vi "Dec_9 - noRamp.vi"() -> ()   [LabVIEW 2020]
uses:
  <vilib>/Utility/error.llb/DialogType.ctl
  <vilib>/Analysis/3filter.llb/Filter Passband Type.ctl
  <vilib>/DAQmx/read.llb/DAQmx Read (Analog 1D DBL NChan 1Samp).vi
  <vilib>/DAQmx/create/channels.llb/DAQmx Create Channel (AI-Voltage-Basic).vi
  <vilib>/DAQmx/configure/timing.llb/DAQmx Timing (Sample Clock).vi
  <vilib>/DAQmx/miscellaneous.llb/DAQmx Fill In Error Info.vi
  <vilib>/Analysis/3filter.llb/Butterworth Filter (DBL).vi
  <vilib>/Utility/file.llb/Write Delimited Spreadsheet (string).vi
  <vilib>/Utility/file.llb/Write Delimited Spreadsheet (DBL).vi
  <vilib>/Analysis/NI_AALBase.lvlib
panel:
  out "Actual Swing":bool
  out "N° step Max":i32
  in  "Choose Automatic Mode":string(combo)
  in  "START":bool
  out "Step Number":i32
  out "Step Counted":bool
  out "Time to Peak (sec)":dbl=200.0
  out "Swing ON Time (sec)":dbl
  in  "Only pre-tension load":bool
  out "Gyro":dynamicdata(graph)
  out "Max Square Wave duration (sec)":dbl
  out "Swing Start Time (sec)":dbl
  out "Time Saved":bool
  out "Pre-Tension Load (N)":dbl
  out "Target Load (N)":dbl=2.0
  out "Release":bool
  out "Pull":bool
  in  "Working Mode":string(combo)
  out "Load Cell":dbl
  in  "Pull CMD":bool
  in  "Release CMD":bool
  out "Load Cell":dynamicdata(graph)
  in  "Motor Torque":dbl(slide) scale=0.0..5.0
  in  "Master Stop":bool
  out "Consumer Loop Speed (ms)":u32
  out "Producer Loop Speed (ms)":u32
  out "Swing":bool
  out "Force Plate":dynamicdata(graph)
  out "Accelerometers":dynamicdata(graph)
  out "Enlapsed Time (sec)":dbl
  # "Choose work mode"
  # "Manual"
  # "Automatic"
  # "Ramp Between-Step Mode"
  # "Ramp Within-Step Mode"
  # "Indicators"
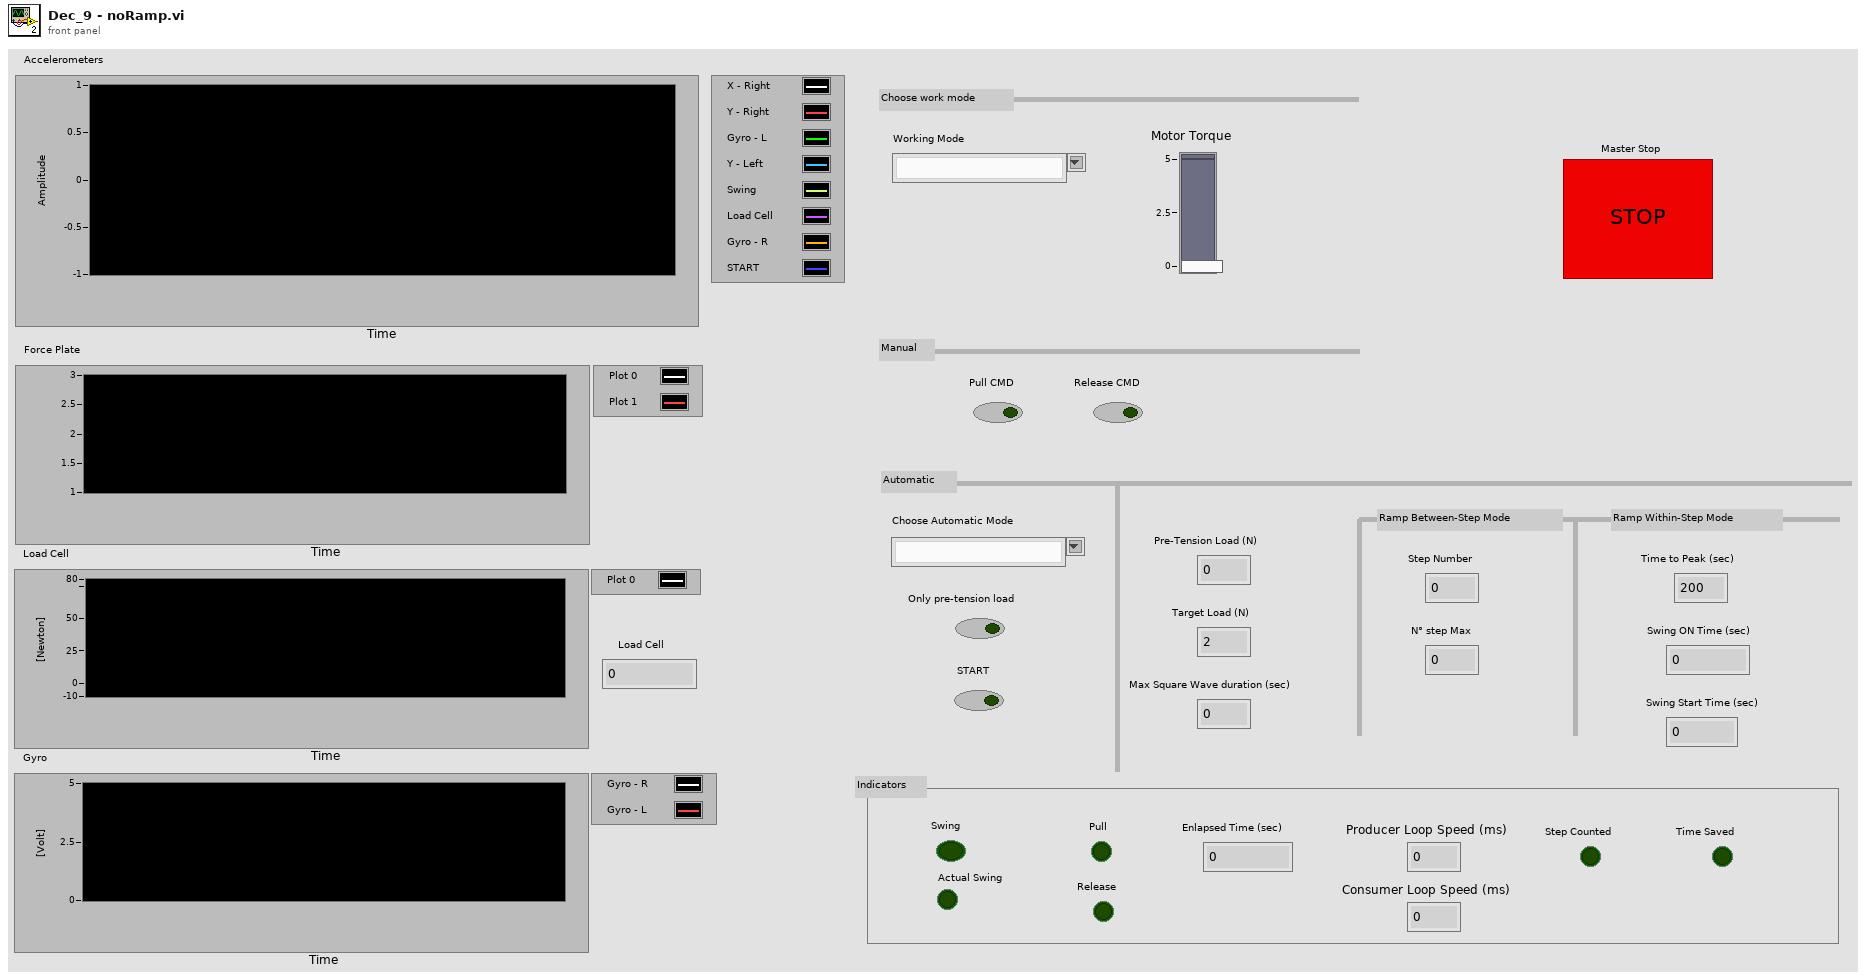
[diagram p1: front panel]
types:
  T1 = typedef "DialogType.ctl" = u16
  T2 = typedef "NI_AALBase.lvlib/Filter Passband Type.ctl" = enum32{"Lowpass", "Highpass", "Bandpass", "Bandstop"}
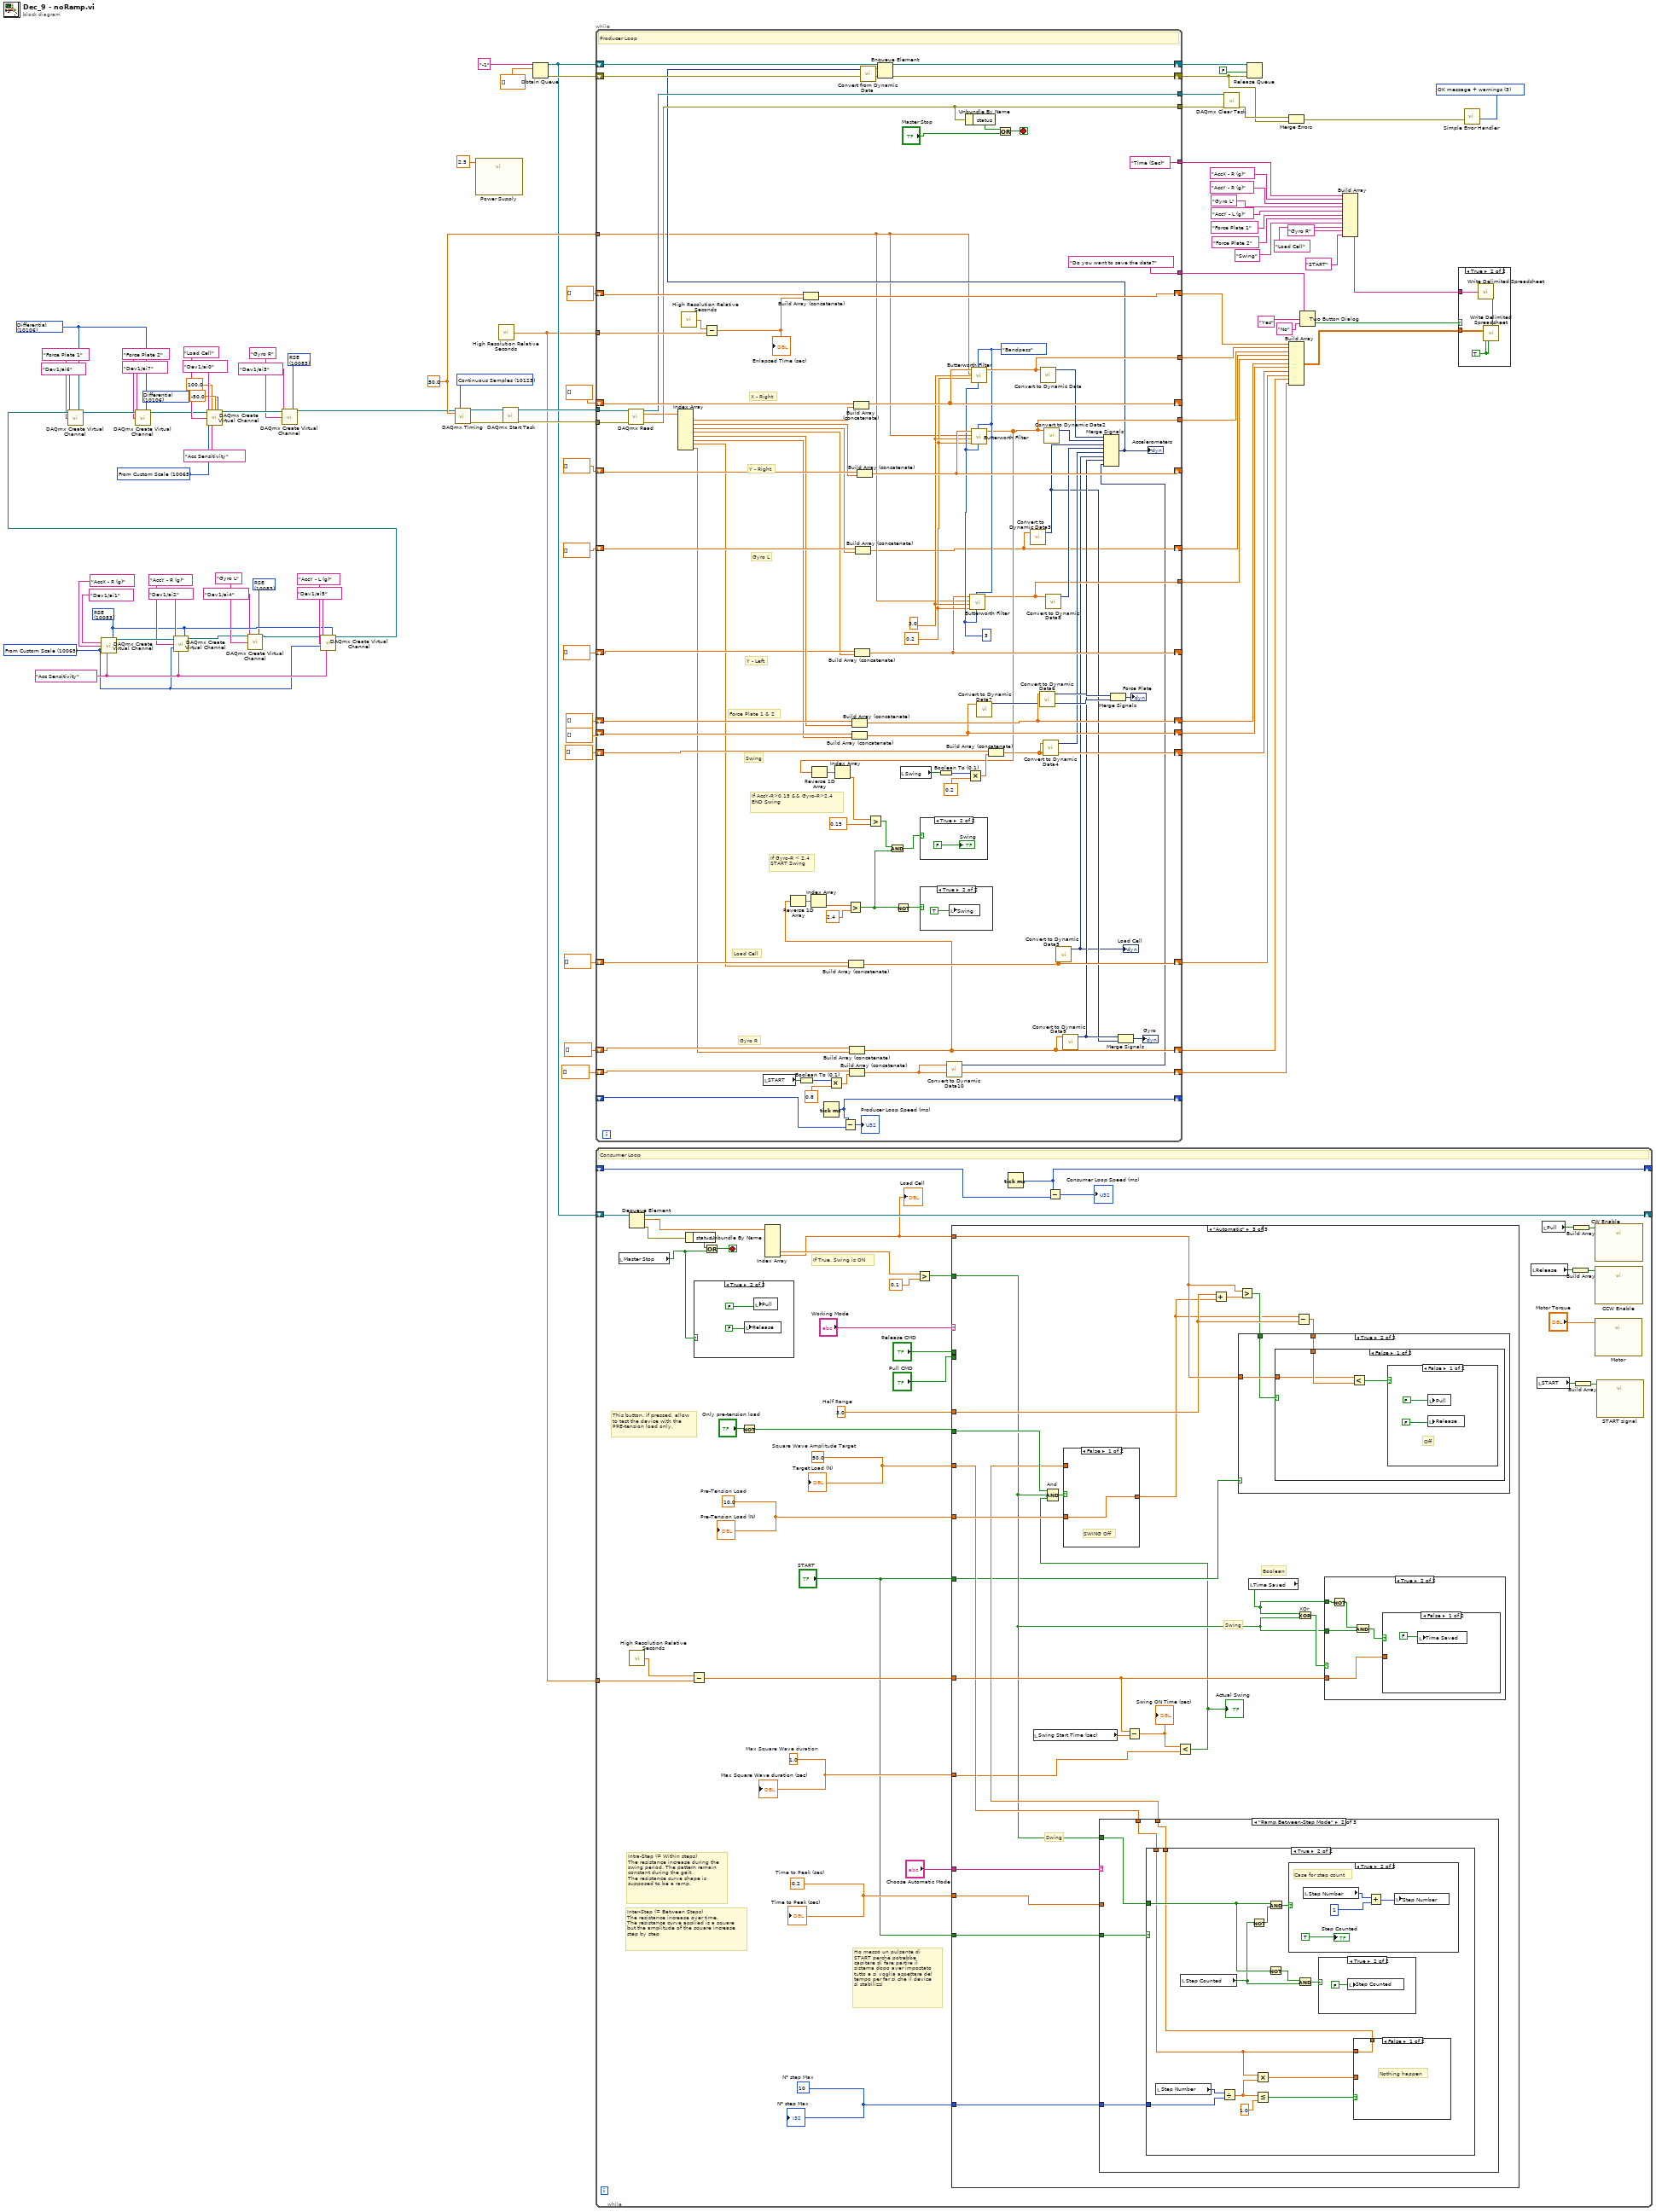
[diagram p0: block diagram]
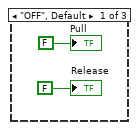
[diagram p3: hidden frame]
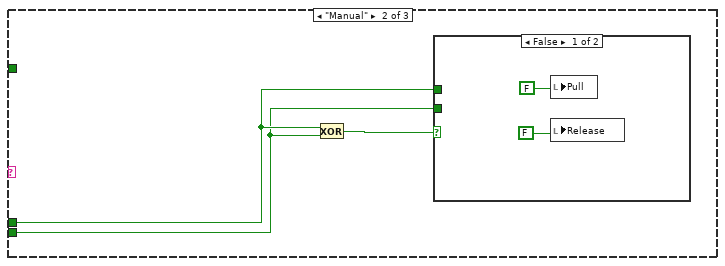
[diagram p4: hidden frame]
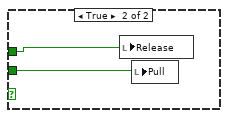
[diagram p5: hidden frame]
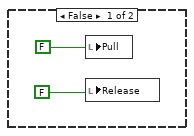
[diagram p6: hidden frame]
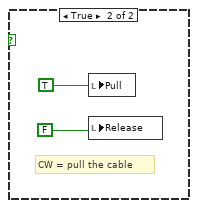
[diagram p7: hidden frame]
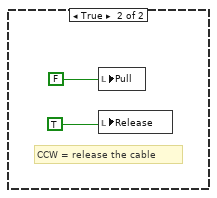
[diagram p8: hidden frame]
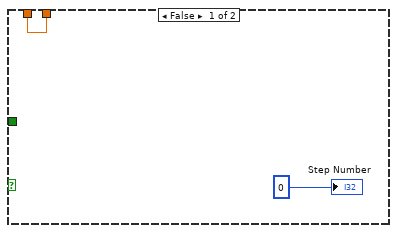
[diagram p10: hidden frame]
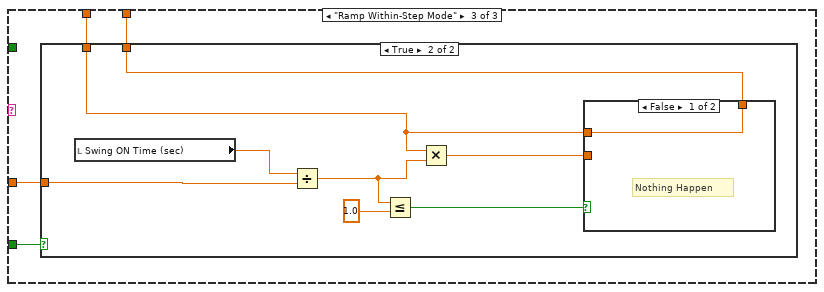
[diagram p14: hidden frame]
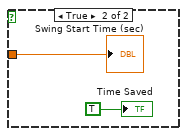
[diagram p18: hidden frame]
diagram:
  w8 = 10083 items=["Default"=-1, "RSE"=10083, "NRSE"=10078, "Differential"=10106, "Pseudodifferential"=12529] ("input terminal configuration")
  w11 = 10106 items=["Default"=-1, "RSE"=10083, "NRSE"=10078, "Differential"=10106, "Pseudodifferential"=12529] ("input terminal configuration")
  w12 = 10083 items=["Default"=-1, "RSE"=10083, "NRSE"=10078, "Differential"=10106, "Pseudodifferential"=12529] ("input terminal configuration")
  w22 = 10065 items=["Volts"=10348, "From Custom Scale"=10065] ("units")
  w37 = T1 3 items=["no dialog", "OK message", "continue or stop message", "OK message + warnings", "continue/stop + warnings"] ("type of dialog (OK msg:1)")
  w27 = 10065 items=["Volts"=10348, "From Custom Scale"=10065] ("units")
  w28 = tag "Acc Sensitivity" ("custom scale name")
  w47 = 10106 items=["Default"=-1, "RSE"=10083, "NRSE"=10078, "Differential"=10106, "Pseudodifferential"=12529] ("input terminal configuration")
  w65 = 10123 items=["Finite Samples"=10178, "Continuous Samples"=10123, "Hardware Timed Single Point"=12522] ("sample mode")
  w60 = 50.0 ("rate")
  w30 = 10083 items=["Default"=-1, "RSE"=10083, "NRSE"=10078, "Differential"=10106, "Pseudodifferential"=12529] ("input terminal configuration")
  n1 = call-poly <vilib>:"DAQmx Create Virtual Channel.vi"("input terminal configuration"=w30, "physical channels"=tag "Dev1/ai1" ("Physical channels"), "name to assign"="AccX - R (g)", "units"=w27, "custom scale name"=w28) -> ("task out"=w59:refnum<k21>)  [unwired: 9 in, 1 out]
  n2 = call-poly <vilib>:"DAQmx Create Virtual Channel.vi"("task in"=w59, "input terminal configuration"=w30, "physical channels"=tag "Dev1/ai2", "name to assign"="AccY - R (g)", "units"=w27, "custom scale name"=w28) -> ("task out"=w7:refnum<k21>)  [unwired: 8 in, 1 out]
  n3 = call-poly <vilib>:"DAQmx Create Virtual Channel.vi"("task in"=w7, "input terminal configuration"=w8, "physical channels"=tag "Dev1/ai4", "name to assign"="Gyro L") -> ("task out"=w6:refnum<k21>)  [unwired: 10 in, 1 out]
  n4 = call-poly <vilib>:"DAQmx Create Virtual Channel.vi"("task in"=w6, "input terminal configuration"=w30, "physical channels"=tag "Dev1/ai5", "name to assign"="AccY - L (g)", "units"=w27, "custom scale name"=w28) -> ("task out"=w58:refnum<k21>)  [unwired: 8 in, 1 out]
  n5 = call-poly <vilib>:"DAQmx Create Virtual Channel.vi"("task in"=w58, "input terminal configuration"=w47, "physical channels"=tag "Dev1/ai6", "name to assign"="Force Plate 1" ("element")) -> ("task out"=w53:refnum<k21>)  [unwired: 10 in, 1 out]
  n6 = call-poly <vilib>:"DAQmx Create Virtual Channel.vi"("task in"=w53, "input terminal configuration"=w47, "physical channels"=tag "Dev1/ai7", "name to assign"="Force Plate 2" ("element")) -> ("task out"=w29:refnum<k21>)  [unwired: 10 in, 1 out]
  n7 = call-poly <vilib>:"DAQmx Create Virtual Channel.vi"("task in"=w29, "maximum value"=100.0, "minimum value"=-50.0, "input terminal configuration"=w11, "physical channels"=tag "Dev1/ai0", "name to assign"="Load Cell", "units"=w22, "custom scale name"=tag "Acc Sensitivity") -> ("task out"=w18:refnum<k21>)  [unwired: 6 in, 1 out]
  n8 = call-poly <vilib>:"DAQmx Create Virtual Channel.vi"("task in"=w18, "input terminal configuration"=w12, "physical channels"=tag "Dev1/ai3", "name to assign"="Gyro R") -> ("task out"=w5:refnum<k21>)  [unwired: 10 in, 1 out]
  n9 = call-poly <vilib>:"DAQmx Timing.vi"("task/channels in"=w5, "sample mode"=w65, "rate"=w60) -> ("task out"=w64:refnum<k21>, "error out"=w63:errorcluster)  [unwired: 11 in]
  n10 = call "Power Supply"("data"=2.5) -> ()  [unwired: 17 in, 2 out]
  n11 = call <vilib>:"High Resolution Relative Seconds.vi"() -> ("relative seconds"=w19:dbl)
  n12 = call <vilib>:"DAQmx Start Task.vi"("task/channels in"=w64, "error in"=w63) -> ("task out"=w62:refnum<k21>, "error out"=w61:errorcluster)  [unwired: 12 in]
  n13 = Obtain Queue(name (unnamed)="-1", element data type=dbl[] []) -> (queue out=w33:refnum<queue>, error out=w42:errorcluster)  [unwired: 3 in, 1 out]
  n14 = while {
    tunnel: w62 -> [w184]
    tunnel: w61 -> [w183]
    tunnel: w19 -> [w181]
    shift-right: [w166] -> w92
    shift-left: dbl[] [] -> [w179]
    shift-right: [w169] -> _
    shift-left: dbl[] [] -> [w178]
    shift-right: [w168] -> _
    shift-left: dbl[] [] -> [w177]
    tunnel: ["Time (Sec)"] -> w68
    tunnel: ["Do you want to save the data?" ("message")] -> w84
    shift-right: [w133] -> w72
    shift-left: dbl[] [] -> [w174]
    shift-right: [w103] -> w4
    shift-left: dbl[] [] -> [w167]
    shift-right: [w157] -> w70
    shift-left: dbl[] [] -> [w160]
    shift-right: [w155] -> w71
    shift-left: dbl[] [] -> [w159]
    tunnel: [w153] -> w74
    tunnel: [w136] -> w73
    shift-right: [w146] -> _
    shift-left: dbl[] [] -> [w145]
    tunnel: [w131] -> w69
    tunnel: w60 -> [w107]
    shift-right: [w138] -> _
    shift-left: _ -> [w137]
    shift-right: [w125] -> w41
    shift-left: w33 -> [w126]
    shift-right: [w123] -> w34
    shift-left: w42 -> [w124]
    tunnel: [w130] -> w39
    tunnel: [w127] -> w38
    shift-right: [w118] -> w25
    shift-left: dbl[] [] -> [w117]
    shift-right: [w112] -> w14
    shift-left: dbl[] [] -> [w115]
    shift-right: [w97] -> w1
    shift-left: dbl[] [] -> [w102]
    stop <- w128 stop-if-true
    w150 = 3 ("order")
    w148 = 0.2 ("low cutoff freq: fl")
    w149 = 3.0 ("high cutoff freq: fh")
    w144 = Filter_Passband_Type."Bandpass" ("filter type")
    # "Gyro L"
    # "Gyro R"
    # "X - Right"
    # "Y - Right"
    # "Y - Left"
    # "Force Plate 1 & 2"
    # "Swing"
    # "Load Cell"
    # "If Gyro-R < 2.4\nSTART Swing"
    # "If AccY-R>0.15 && Gyro-R>2.4\nEND Swing"
    # "Producer Loop"
    n15 = call-poly <vilib>:"DAQmx Read.vi"("task/channels in"=w184, "error in"=w183) -> ("task out"=w130:refnum<k21>, "data"=w122:dbl[], "error out"=w127:errorcluster)  [unwired: 11 in]
    n16 = Index Array(array=w122) -> (element #1=w143:dbl, element #2=w142:dbl, element #3=w141:dbl, element #4=w140:dbl, element #5=w151:dbl, element #6=w152:dbl, element #7=w116:dbl, element #8=w114:dbl)  [unwired: 8 in]
    n17 = call <vilib>:"High Resolution Relative Seconds.vi"() -> ("relative seconds"=w182:dbl)
    n18 = Subtract(x=w182, y=w181) -> (x-y=w180:dbl)
    "Enlapsed Time (sec)" <- w180
    n19 = local read "START"() -> (w98:bool)
    n20 = Boolean To (0,1)(Boolean=w98) -> (0, 1=w101:i16)
    n21 = Build Array (concatenate)(w179, w180) -> (w166:dbl[])
    n22 = Tick Count (ms)() -> (millisecond timer value=w138:u32)
    n23 = Multiply(x=w101, y=0.8) -> (x*y=w99:dbl)
    n24 = Subtract(x=w138, y=w137) -> (x-y=→"Producer Loop Speed (ms)":u32)
    n25 = Build Array (concatenate)(w117, w116) -> (w118:dbl[])
    n26 = Build Array (concatenate)(w115, w114) -> (w112:dbl[])
    n27 = Reverse 1D Array(array=w112) -> (reversed array=w162:dbl[])
    n28 = Index Array(array=w162) -> (element=w161:dbl)  [unwired: 1 in]
    n29 = Greater?(x=w161, y=2.4) -> (0:w108:bool)
    n30 = Build Array (concatenate)(w102, w99) -> (w97:dbl[])
    n31 = Build Array (concatenate)(w160, w151) -> (w157:dbl[])
    n32 = Build Array (concatenate)(w159, w152) -> (w155:dbl[])
    n33 = Build Array (concatenate)(w178, w143) -> (w169:dbl[])
    n34 = Build Array (concatenate)(w145, w140) -> (w146:dbl[])
    n35 = Build Array (concatenate)(w167, w141) -> (w103:dbl[])
    n36 = Build Array (concatenate)(w177, w142) -> (w168:dbl[])
    n37 = Not(x=w108) -> (.not. x?=w109:bool)
    n38 = local read "Swing"() -> (w95:bool)
    n39 = case shown="True" w109 {
      frame False {
      }
      frame True {
        n40 = local write "Swing"(TRUE) -> ()
      }
    }
    n41 = Boolean To (0,1)(Boolean=w95) -> (0, 1=w172:i16)
    n42 = call "Convert to Dynamic Data10"("Array"=w97) -> ("Dynamic Data Type"=w96:dynamicdata)  [unwired: 3 in]
    n43 = Unbundle By Name(w127) -> ("status"=w129:bool)
    n44 = Multiply(x=w172, y=0.2) -> (x*y=w173:dbl)
    n45 = call-poly <vilib>:"Butterworth Filter.vi"("order"=w150, "filter type"=w144, "low cutoff freq: fl"=w148, "high cutoff freq: fh"=w149, "sampling freq: fs"=w107, "X"=w146) -> ("Filtered X"=w131:dbl[])  [unwired: 2 in, 1 out]
    n46 = call-poly <vilib>:"Butterworth Filter.vi"("order"=w150, "filter type"=w144, "low cutoff freq: fl"=w148, "high cutoff freq: fh"=w149, "sampling freq: fs"=w107, "X"=w169) -> ("Filtered X"=w153:dbl[])  [unwired: 2 in, 1 out]
    n47 = call-poly <vilib>:"Butterworth Filter.vi"("order"=w150, "filter type"=w144, "low cutoff freq: fl"=w148, "high cutoff freq: fh"=w149, "sampling freq: fs"=w107, "X"=w168) -> ("Filtered X"=w136:dbl[])  [unwired: 2 in, 1 out]
    n48 = Reverse 1D Array(array=w136) -> (reversed array=w170:dbl[])
    n49 = Index Array(array=w170) -> (element=w135:dbl)  [unwired: 1 in]
    n50 = Greater?(x=w135, y=0.15) -> (0:w110:bool)
    n51 = And(x=w110, y=w108) -> (x .and. y?=w111:bool)
    n52 = case shown="True" w111 {
      frame False {
      }
      frame True {
        "Swing" <- FALSE
      }
    }
    n53 = call "Convert to Dynamic Data7"("Array"=w155) -> ("Dynamic Data Type"=w154:dynamicdata)  [unwired: 3 in]
    n54 = Build Array (concatenate)(w174, w173) -> (w133:dbl[])
    n55 = Or(x=w129, y="Master Stop") -> (x .or. y?=w128:bool)
    n56 = call "Convert to Dynamic Data3"("Array"=w103) -> ("Dynamic Data Type"=w105:dynamicdata)  [unwired: 3 in]
    n57 = call "Convert to Dynamic Data6"("Array"=w157) -> ("Dynamic Data Type"=w156:dynamicdata)  [unwired: 3 in]
    n58 = call "Convert to Dynamic Data"("Array"=w153) -> ("Dynamic Data Type"=w165:dynamicdata)  [unwired: 3 in]
    n59 = call "Convert to Dynamic Data4"("Array"=w133) -> ("Dynamic Data Type"=w132:dynamicdata)  [unwired: 3 in]
    n60 = call "Convert to Dynamic Data2"("Array"=w136) -> ("Dynamic Data Type"=w164:dynamicdata)  [unwired: 3 in]
    n61 = call "Convert to Dynamic Data8"("Array"=w131) -> ("Dynamic Data Type"=w147:dynamicdata)  [unwired: 3 in]
    n62 = call "Convert to Dynamic Data5"("Array"=w118) -> ("Dynamic Data Type"=w104:dynamicdata)  [unwired: 3 in]
    "Load Cell" <- w104
    n63 = call "Convert to Dynamic Data9"("Array"=w112) -> ("Dynamic Data Type"=w113:dynamicdata)  [unwired: 3 in]
    n64 = Merge Signals(w165, w164, w105, w147, w132, w104, w113, w96) -> (w120:dynamicdata)
    "Accelerometers" <- w120
    n65 = call "Convert from Dynamic Data"("Dynamic Data Type"=w120) -> ("Array"=w119:dbl[])  [unwired: 3 in]
    n66 = Enqueue Element(queue=w126, element=w119, error in (no error)=w124) -> (queue out=w125:refnum<queue>, error out=w123:errorcluster)  [unwired: 1 in, 1 out]
    n67 = Merge Signals(w156, w154) -> (→"Force Plate":dynamicdata)
    n68 = Merge Signals(w113, w105) -> (→"Gyro":dynamicdata)
  }
  n69 = while {
    shift-right: [w222] -> _
    shift-left: w33 -> [w223]
    shift-right: [w219] -> _
    shift-left: _ -> [w220]
    tunnel: w19 -> [w197]
    stop <- w217 stop-if-true
    w190 = 10  # N° step Max
    w192 = 0.2  # Time to Peak (sec)
    w195 = 1.0  # Max Square Wave duration
    w199 = 3.0  # Half Range
    w200 = 10.0  # Pre-Tension Load
    w201 = 50.0  # Square Wave Amplitude Target
    # "Ho messo un pulsante di \nSTART perchè potrebbe\ncapitare di fare partire il \nsistema dopo aver impostato \ntutto e si voglia aspettare del \ntempo per far si che il device\nsi stabilizzi"
    # "Inter-Step (= Between Steps)\nThe resistance increase over time.\nThe resistance curve applied is a square\nbut the amplitude of the square increase \nstep by step"
    # "Intra-Step (= Within steps) \nThe resistance increase during the\nswing period. The pattern remain \nconstant during the gait.\nThe resistance curve shape is \nsupposed to be a ramp."
    # "This button, if pressed, allow\nto test the device with the\nPRE-tension load only."
    # "If True, Swing is ON"
    # "Consumer Loop"
    n70 = local read "Master Stop"() -> (w202:bool)
    n71 = Dequeue Element(queue=w223) -> (queue out=w222:refnum<queue>, element=w215:dbl[], error out=w216:errorcluster)  [unwired: 2 in, 1 out]
    n72 = call <vilib>:"High Resolution Relative Seconds.vi"() -> ("relative seconds"=w198:dbl)
    n73 = Unbundle By Name(w216) -> ("status"=w218:bool)
    n74 = Subtract(x=w198, y=w197) -> (x-y=w196:dbl)
    n75 = case shown="True" w202 {
      frame False {
      }
      frame True {
        n76 = local write "Release"(FALSE) -> ()
        n77 = local write "Pull"(FALSE) -> ()
      }
    }
    n78 = Or(x=w218, y=w202) -> (x .or. y?=w217:bool)
    n79 = Not(x="Only pre-tension load") -> (.not. x?=w193:bool)
    n80 = Index Array(array=w215) -> (element #5=w214:dbl, element #6=w212:dbl)  [unwired: 6 in, 4 out]
    "Load Cell" <- w212
    n81 = Greater?(x=w214, y=0.1) -> (0:w203:bool)
    n82 = case shown="\"Automatic\"" "Working Mode" {
      tunnel: w212 -> [_ _ w258]
      tunnel: "Release CMD" -> [_ w229 _]
      tunnel: "Pull CMD" -> [_ w228 _]
      tunnel: w203 -> [_ _ w241]
      tunnel: w201 -> [_ _ w246]
      tunnel: w200 -> [_ _ w253]
      tunnel: w199 -> [_ _ w257]
      tunnel: w196 -> [_ _ w248]
      tunnel: w195 -> [_ _ w235]
      tunnel: w193 -> [_ _ w249]
      tunnel: w192 -> [_ _ w244]
      tunnel: "START" -> [_ _ w240]
      tunnel: "Choose Automatic Mode" -> [_ _ w242]
      tunnel: w190 -> [_ _ w239]
      tunnel: "START" -> [_ _ w238]
      frame "OFF", Default {
        "Pull" <- FALSE
        "Release" <- FALSE
      }
      frame "Manual" {
        n83 = Exclusive Or(1:w228, 2:w229) -> (0:w230:bool)
        n84 = case shown="False" w230 {
          tunnel: w229 -> [_ w233]
          tunnel: w228 -> [_ w234]
          frame False {
            n85 = local write "Pull"(FALSE) -> ()
            n86 = local write "Release"(FALSE) -> ()
          }
          frame True {
            n87 = local write "Release"(w233) -> ()
            n88 = local write "Pull"(w234) -> ()
          }
        }
      }
      frame "Automatic" {
        # "Swing"
        # "Boolean"
        # "Swing"
        n89 = local read "Swing Start Time (sec)"() -> (w247:dbl)
        n90 = case shown="\"Ramp Between-Step Mode\"" w242 {
          tunnel: w246 -> [w273 w276 w303]
          tunnel: [w273 w275 w304] -> w245
          tunnel: w244 -> [_ _ w305]
          tunnel: w241 -> [_ w278 _]
          tunnel: w240 -> [_ w277 w302]
          tunnel: w239 -> [_ w274 _]
          frame "No Ramp", Default {
            # "If the ramp mode is OFF, \nnothing happen. \nThe SWA target remain the same."
          }
          frame "Ramp Between-Step Mode" {
            n91 = case shown="True" w277 {
              tunnel: w278 -> [_ w293]
              tunnel: w276 -> [w279 w282]
              tunnel: [w279 w284] -> w275
              tunnel: w274 -> [_ w287]
              frame False {
                "Step Number" <- 0
              }
              frame True {
                n92 = local read "Step Number"() -> (w288:i32)
                n93 = local read "Step Counted"() -> (w291:bool)
                n94 = Divide(x=w288, y=w287) -> (x/y=w283:dbl)
                n95 = Not(x=w291) -> (.not. x?=w292:bool)
                n96 = Multiply(x=w282, y=w283) -> (x*y=w281:dbl)
                n97 = Less Or Equal?(x=w283, y=1.0) -> (x <= y?=w285:bool)
                n98 = Not(x=w293) -> (.not. x?=w289:bool)
                n99 = And(x=w293, y=w292) -> (x .and. y?=w294:bool)
                n100 = case shown="True" w294 {
                  frame False {
                  }
                  frame True {
                    # "Case for step count"
                    n101 = local read "Step Number"() -> (w300:i32)
                    n102 = Add(x=w300, y=1) -> (x+y=w299:i32)
                    n103 = local write "Step Number"(w299) -> ()
                    "Step Counted" <- TRUE
                  }
                }
                n104 = And(x=w289, y=w291) -> (x .and. y?=w290:bool)
                n105 = case shown="True" w290 {
                  frame False {
                  }
                  frame True {
                    n106 = local write "Step Counted"(FALSE) -> ()
                  }
                }
                n107 = case shown="False" w285 {
                  tunnel: w282 -> [w295 _]
                  tunnel: [w295 w296] -> w284
                  tunnel: w281 -> [_ w296]
                  frame False {
                    # "Nothing happen"
                  }
                  frame True {
                  }
                }
              }
            }
          }
          frame "Ramp Within-Step Mode" {
            n108 = case shown="True" w302 {
              tunnel: w305 -> [_ w313]
              tunnel: [w306 w311] -> w304
              tunnel: w303 -> [w306 w307]
              frame False {
              }
              frame True {
                n109 = local read "Swing ON Time (sec)"() -> (w314:dbl)
                n110 = Divide(x=w314, y=w313) -> (x/y=w309:dbl)
                n111 = Less Or Equal?(x=w309, y=1.0) -> (x <= y?=w308:bool)
                n112 = Multiply(x=w307, y=w309) -> (x*y=w312:dbl)
                n113 = case shown="False" w308 {
                  tunnel: w312 -> [_ w316]
                  tunnel: [w315 w316] -> w311
                  tunnel: w307 -> [w315 _]
                  frame False {
                    # "Nothing Happen"
                  }
                  frame True {
                  }
                }
              }
            }
          }
        }
        n114 = Subtract(x=w248, y=w247) -> (x-y=w236:dbl)
        "Swing ON Time (sec)" <- w236
        n115 = Less?(x=w236, y=w235) -> (x < y?=w237:bool)
        "Actual Swing" <- w237
        n116 = Compound Arithmetic op=AND "And"(w249, w241, w237) -> (w243:bool)
        n117 = case shown="False" w243 {
          tunnel: w245 -> [_ w326]
          tunnel: w253 -> [w325 _]
          tunnel: [w325 w326] -> w252
          frame False {
            # "SWING Off"
          }
          frame True {
            # "SWING ON"
          }
        }
        n118 = Add(x=w257, y=w252) -> (x+y=w255:dbl)
        n119 = Greater?(x=w258, y=w255) -> (0:w256:bool)
        n120 = local read "Time Saved"() -> (w250:bool)
        n121 = Subtract(x=w252, y=w257) -> (x-y=w254:dbl)
        n122 = case shown="True" w238 {
          tunnel: w258 -> [_ w263]
          tunnel: w256 -> [_ w262]
          tunnel: w254 -> [_ w261]
          frame False {
            n123 = local write "Pull"(FALSE) -> ()
            n124 = local write "Release"(FALSE) -> ()
          }
          frame True {
            n125 = case shown="False" w262 {
              tunnel: w263 -> [w265 _]
              tunnel: w261 -> [w266 _]
              frame False {
                n126 = Less?(x=w265, y=w266) -> (x < y?=w264:bool)
                n127 = case shown="False" w264 {
                  frame False {
                    # "Off"
                    n128 = local write "Pull"(FALSE) -> ()
                    n129 = local write "Release"(FALSE) -> ()
                  }
                  frame True {
                    # "CW = pull the cable"
                    n130 = local write "Pull"(TRUE) -> ()
                    n131 = local write "Release"(FALSE) -> ()
                  }
                }
              }
              frame True {
                # "CCW = release the cable"
                n132 = local write "Pull"(FALSE) -> ()
                n133 = local write "Release"(TRUE) -> ()
              }
            }
          }
        }
        n134 = Exclusive Or "XOr"(1:w241, 2:w250) -> (0:w251:bool)
        n135 = case shown="True" w251 {
          tunnel: w248 -> [_ w321]
          tunnel: w250 -> [_ w317]
          tunnel: w241 -> [_ w319]
          frame False {
          }
          frame True {
            n136 = Not(x=w317) -> (.not. x?=w318:bool)
            n137 = And(x=w318, y=w319) -> (x .and. y?=w320:bool)
            n138 = case shown="False" w320 {
              tunnel: w321 -> [_ w324]
              frame False {
                n139 = local write "Time Saved"(FALSE) -> ()
              }
              frame True {
                "Swing Start Time (sec)" <- w324
                "Time Saved" <- TRUE
              }
            }
          }
        }
      }
    }
    n140 = Tick Count (ms)() -> (millisecond timer value=w219:u32)
    n141 = Subtract(x=w219, y=w220) -> (x-y=→"Consumer Loop Speed (ms)":u32)
    n142 = local read "Release"() -> (w206:bool)
    n143 = local read "START"() -> (w188:bool)
    n144 = local read "Pull"() -> (w207:bool)
    n145 = Build Array(w206) -> (w208:bool[])
    n146 = Build Array(w207) -> (w209:bool[])
    n147 = Build Array(w188) -> (w187:bool[])
    n148 = call "Motor"("data"="Motor Torque") -> ()  [unwired: 17 in, 2 out]
    n149 = call "CW Enable"("data"=w209) -> ()  [unwired: 17 in, 2 out]
    n150 = call "CCW Enable"("data"=w208) -> ()  [unwired: 17 in, 2 out]
    n151 = call "START signal"("data"=w187) -> ()  [unwired: 17 in, 2 out]
    "Target Load (N)" <- w201
    "Pre-Tension Load (N)" <- w200
    "Max Square Wave duration (sec)" <- w195
    "Time to Peak (sec)" <- w192
    "N° step Max" <- w190
  }
  n152 = call <vilib>:"DAQmx Clear Task.vi"("task in"=w39, "error in"=w38) -> ("error out"=w35:errorcluster)  [unwired: 13 out]
  n153 = Release Queue(queue=w41, force destroy? (F)=FALSE, error in (no error)=w34) -> ()  [unwired: 3 out]
  n154 = Merge Errors(w35, w34) -> (w36:errorcluster)
  n155 = Build Array(w92, w74, w73, w4, w69, w70, w71, w72, w25, w14, w1) -> (w91:dbl[][])
  n156 = Two Button Dialog(message=w84, 1:"No" ("F button name (\"Cancel\")"), 2:"Yes" ("T button name (\"OK\")")) -> (T button?=w87:bool)
  n157 = Build Array(w68, "AccX - R (g)", "AccY - R (g)", "Gyro L", "AccY - L (g)", "Force Plate 1" ("element"), "Force Plate 2" ("element"), "Swing" ("element"), "Load Cell" ("element"), "Gyro R" ("element"), "START" ("element")) -> (w90:string[])
  n158 = case shown="True" w87 {
    tunnel: w91 -> [_ w330]
    tunnel: w90 -> [_ w329]
    frame False {
    }
    frame True {
      w328 = TRUE ("transpose? (no:F)")
      n159 = call-poly <vilib>:"Write Delimited Spreadsheet.vi"("1D data"=w329) -> ("new file path (Not A Path if cancelled)"=w327:path)  [unwired: 13 in, 1 out]
      n160 = call-poly <vilib>:"Write Delimited Spreadsheet.vi"("file path (dialog if empty)"=w327, "2D data"=w330, "append to file? (new file:F)"=w328, "transpose? (no:F)"=w328) -> ()  [unwired: 10 in, 2 out]
    }
  }
  n161 = call <vilib>:"Simple Error Handler.vi"("type of dialog (OK msg:1)"=w37, "error in (no error)"=w36) -> ()  [unwired: 8 out]
